vi "configure gating.vi"(8 "error in (no error)":errorcluster, 9 "GatingMode":u32(ring) items=["FreeRunning", "TriggerRising", "TriggerFalling", "TriggerBoth", "GatedHigh", "GatedLow"], 10 "Board":u16, 11 "identifier":string) -> (0 "error out":errorcluster, 3 "function return":u32)   [LabVIEW 2015, in "XGL_DPP.lvlib"]
doc: "EXTERN DECLSPEC uint32_t CALL_CONV configure_gating(const char * identifier, uint16_t Board, const GatingMode GatingMode);"
uses:
  DANTE/DANTE-v2.0.8.9/DANTE v2.0.8.9/Examples/Labview2013/libs/XGL_DPP.lvlib
  DANTE/DANTE-v2.0.8.9/DANTE v2.0.8.9/Acquisition Software/GUI_DANTE_x64/XGL_DPP.dll
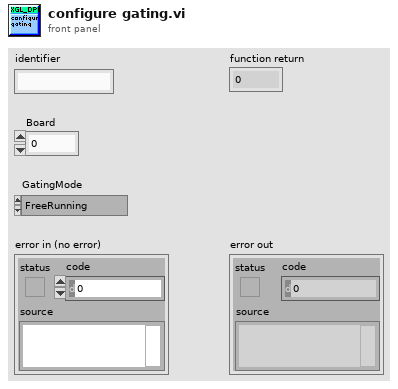
[diagram p1: front panel]
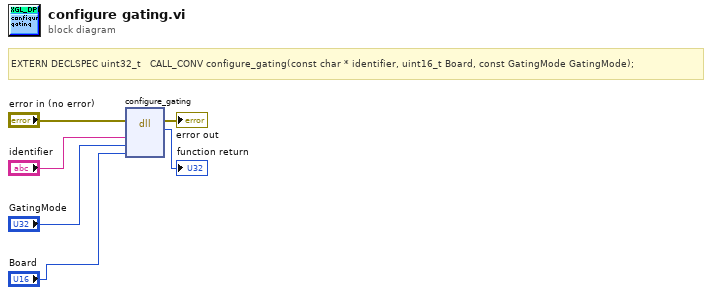
[diagram p0: block diagram]
diagram:
  # "EXTERN DECLSPEC uint32_t   CALL_CONV configure_gating(const char * identifier, uint16_t Board, const GatingMode GatingMode);"
  n1 = dll-call lib="D:/DANTE/DANTE-v2.0.8.9/DANTE v2.0.8.9/Acquisition Software/GUI_DANTE_x64/XGL_DPP.*" fn="configure_gating"(error in="error in (no error)", "identifier"="identifier", "GatingMode"="GatingMode", "Board"="Board") -> (error out=→"error out":errorcluster, "return type"=→"function return":u32)  [unwired: 5 in, 1 out]
